vi "Test XY Graph with TipStrip.vi"() -> ()   [LabVIEW 2021, in "XY Graph Add-Ons.lvlib"]
uses:
  XY Graph/XY Graph Add-Ons.lvlib
  XY Graph/XY Graph Refnum.ctl
  XY Graph/XY Graph Event.ctl
  <vilib>/Utility/miscctls.llb/LVPoint32TypeDef.ctl
  4bea80b7-e27f-4baa-81f5-8c3dcb08d727.vi
panel:
  out "XY Graph TipStrip":string
  out "XY Graph":cluster{dbl[], dbl[]}[](graph)
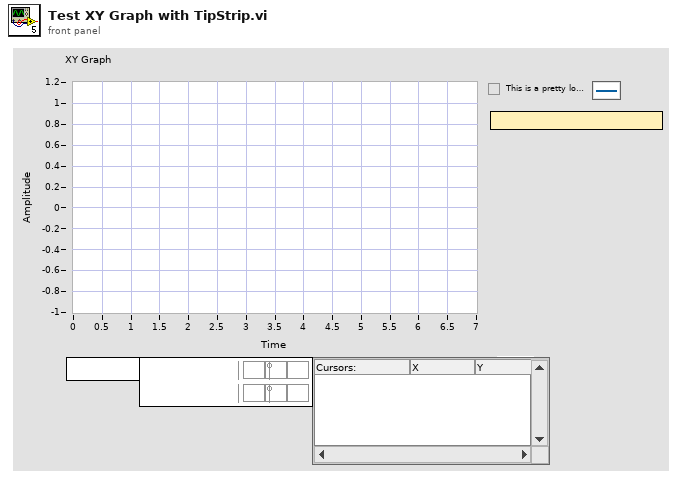
[diagram p1: front panel]
types:
  T1 = cluster{"XY Graph TipStrip":refnum<event-registration>}
  T2 = typedef "XY Graph Add-Ons.lvlib/XY Graph Event.ctl" = cluster{"Item Tag":string, "XY Graph Refnum":refnum<vi>, "Coords":T3, "Item Path":string}
  T3 = typedef "LVPoint32TypeDef.ctl" = cluster{"Horizontal":i32, "Vertical":i32}
  T4 = typedef "XY Graph Add-Ons.lvlib/XY Graph Tool Panels Visibility.ctl" = cluster{"Scale Legend Vis":bool, "X-Scrollbar Vis":bool, "Cursor Panel Vis":bool, "Graph Palette Vis":bool}
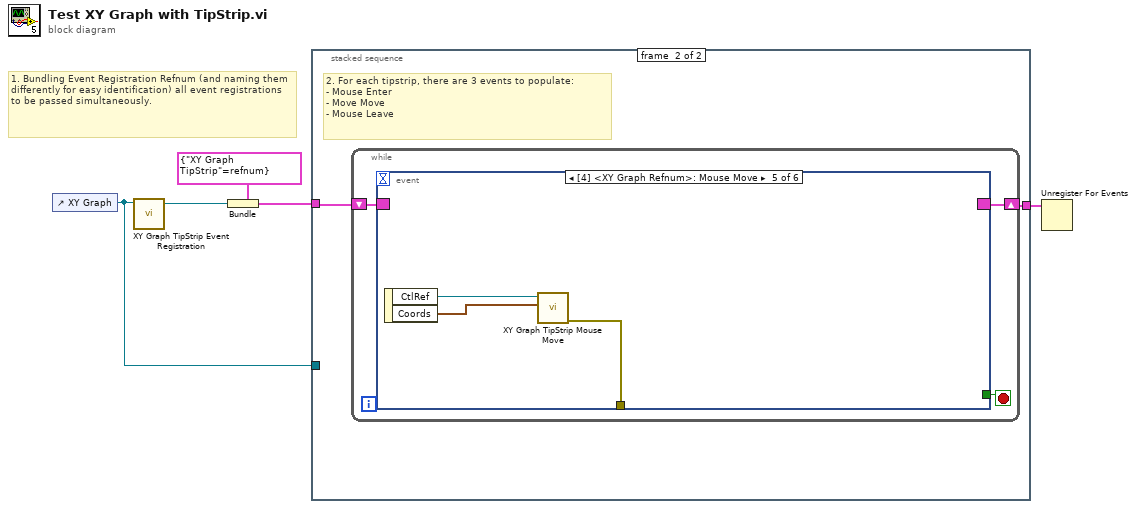
[diagram p0: block diagram]
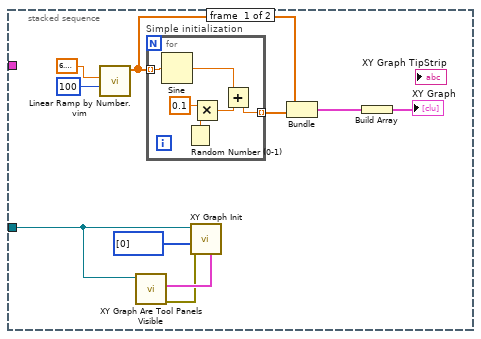
[diagram p2: hidden frame]
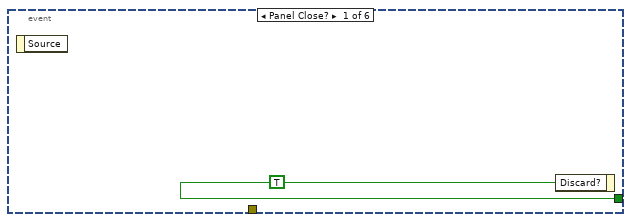
[diagram p3: hidden frame]
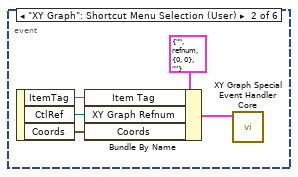
[diagram p4: hidden frame]
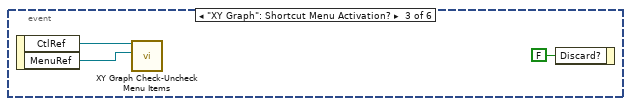
[diagram p5: hidden frame]
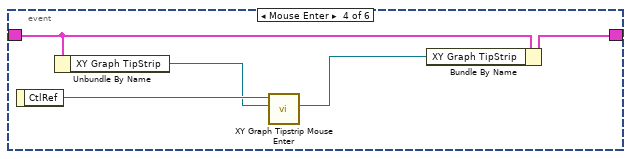
[diagram p6: hidden frame]
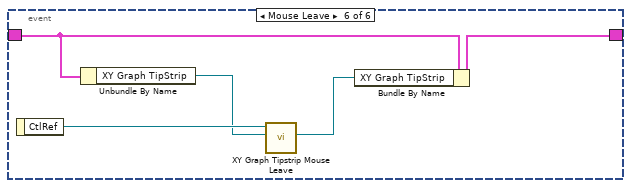
[diagram p7: hidden frame]
diagram:
  # "1. Bundling Event Registration Refnum (and naming them differently for easy identification) all event registrations to be passed simultaneously."
  n1 = control-ref of="XY Graph"() -> (w2:refnum<vi>)
  n2 = call "XY Graph TipStrip Event Registration.vi"("XY Graph Refnum"=w2) -> ("Event Registration Refnum"=w5:refnum<event-registration>)  [unwired: 8 in, 2 out]
  n3 = Bundle(cluster=T1 {"XY Graph TipStrip"=refnum} ("Event Registration Refnums"), "XY Graph TipStrip"=w5) -> (w3:T1)
  n4 = stacked-sequence {
    tunnel: [_ w23] -> w4
    tunnel: w3 -> [_ w22]
    tunnel: w2 -> [w11 _]
    frame #0 {
      n5 = call "Linear Ramp by Number.vim"("# Steps (1)"=100, "End (1)"=6.283185307179586) -> ("Ramp"=w6:dbl[])  [unwired: 7 in, 2 out]
      n6 = call "XY Graph Are Tool Panels Visible.vi"("XY Graph Ref"=w11) -> ("Error Out"=w9:errorcluster, "Graph Tool Panels Visibility"=w10:T4)  [unwired: 7 in, 2 out]
      n7 = for "Simple initialization" {
        tunnel: [w16] -> w14 mode=indexing
        tunnel: w6 -> [w21] mode=indexing
        n8 = Sine(x=w21) -> (sin(x)=w18:dbl)
        n9 = Random Number (0-1)() -> (number: 0 to 1=w20:dbl)
        n10 = Multiply(x=0.1, y=w20) -> (x*y=w17:dbl)
        n11 = Add(x=w18, y=w17) -> (x+y=w16:dbl)
      }
      n12 = call "XY Graph Init.vi"("Graph Tool Panels Visibility"=w10, "Error In"=w9, "Plots to Skip (none)"=i32[] [0], "XYGraph in"=w11) -> ()  [unwired: 7 in, 1 out]
      n13 = Bundle("Ramp"=w6, w14) -> (w15:cluster{"Ramp":dbl[], dbl[]})  [unwired: 1 in]
      n14 = Build Array(w15) -> (→"XY Graph":cluster{"Ramp":dbl[], dbl[]}[])
    }
    frame #1 {
      # "2. For each tipstrip, there are 3 events to populate:\n- Mouse Enter\n- Move Move\n- Mouse Leave"
      n15 = while {
        shift-right: [w24] -> w23
        shift-left: w22 -> [w26]
        stop <- w25 stop-if-true
        n16 = event shown="[4] <XY Graph Refnum>: Mouse Move" {
          selector: w26 -> [_ _ _ w38 _ w45]
          dyn-events: [_ _ _ w40 _ w44] -> w24
          timeout: _ -> [_ _ _ _ _ _]
          tunnel: [w27 _ _ _ _ _] -> w25
          tunnel: [_ _ _ _ w41 _] -> _
          event Panel Close? {
            w27 = TRUE ("Discard?")
            n17 = event-data() -> ()  [unwired: 1 in, 1 out]
            n18 = event-data("Discard?"=w27) -> ()  [unwired: 1 in, 1 out]
          }
          event "XY Graph": Shortcut Menu Selection (User) {
            n19 = event-data() -> ("ItemTag"=w30:string, "CtlRef"=w29:refnum<vi>, "Coords"=w28:T3)  [unwired: 1 in]
            n20 = Bundle By Name(cluster=T2 {"Item Tag"="", "XY Graph Refnum"=refnum, "Coords"={"Horizontal"=0, "Vertical"=0}, "Item Path"=""} ("XY Graph Event"), "Item Tag"=w30, "XY Graph Refnum"=w29, "Coords"=w28) -> (w31:T2)
            n21 = call "XY Graph Special Event Handler Core.vi"("XY Graph Event"=w31) -> ()  [unwired: 6 in, 5 out]
          }
          event "XY Graph": Shortcut Menu Activation? {
            n22 = event-data() -> ("CtlRef"=w34:refnum<vi>, "MenuRef"=w33:refnum<k9>)  [unwired: 1 in]
            n23 = call "XY Graph Check-Uncheck Menu Items.vi"("Menu in"=w33, "XY Graph Refnum"=w34) -> ()  [unwired: 6 in, 4 out]
            n24 = event-data("Discard?"=FALSE) -> ()  [unwired: 1 in, 1 out]
          }
          event Mouse Enter {
            n25 = event-data() -> ("CtlRef"=w39:refnum<vi>)  [unwired: 1 in]
            n26 = Unbundle By Name(w38) -> ("XY Graph TipStrip"=w37:refnum<event-registration>)
            n27 = call "XY Graph Tipstrip Mouse Enter.vi"("Event Registration Refnum"=w37, "XY Graph Refnum"=w39) -> ("Event Registration Refnum"=w36:refnum<event-registration>)  [unwired: 8 in, 1 out]
            n28 = Bundle By Name(cluster=w38, "XY Graph TipStrip"=w36) -> (w40:T1)
          }
          event Mouse Move {
            n29 = event-data() -> ("CtlRef"=w43:refnum<vi>, "Coords"=w42:T3)  [unwired: 1 in]
            n30 = call "XY Graph TipStrip Mouse Move.vi"("Coords"=w42, "XY Graph Refnum"=w43) -> ("Error Out"=w41:errorcluster)  [unwired: 7 in, 2 out]
          }
          event Mouse Leave {
            n31 = event-data() -> ("CtlRef"=w48:refnum<vi>)  [unwired: 1 in]
            n32 = Unbundle By Name(w45) -> ("XY Graph TipStrip"=w47:refnum<event-registration>)
            n33 = call "XY Graph Tipstrip Mouse Leave.vi"("Event Registration Refnum"=w47, "XY Graph Refnum"=w48) -> ("Event Registration Refnum"=w46:refnum<event-registration>)  [unwired: 8 in, 1 out]
            n34 = Bundle By Name(cluster=w45, "XY Graph TipStrip"=w46) -> (w44:T1)
          }
        }
      }
    }
  }
  n35 = Unregister For Events(event registration refnum=w4) -> ()  [unwired: 1 in, 1 out]
